vi "Values.vi"(8 "error in (no error)":errorcluster, 11 "VariantAttribute in":refnum<class "MapImp.lvclass">) -> (0 "error out":errorcluster, 1 "Values":refnum<class>[](array[class]), 3 "VariantAttribute out":refnum<class "MapImp.lvclass">)   [LabVIEW 2013, in "LapDog.Collections.v_.Maps.lvlib" / "MapImp.lvclass"]
doc: "Returns a copy of all values in the map."
uses:
  MapImp.lvclass
  MapImp.lvclass/MapImp.ctl
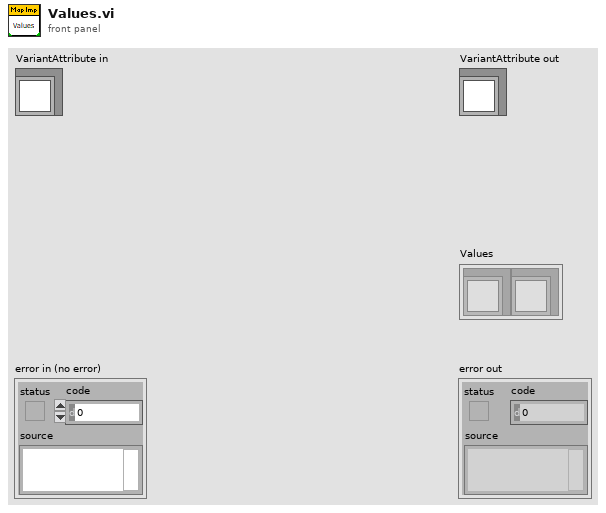
[diagram p1: front panel]
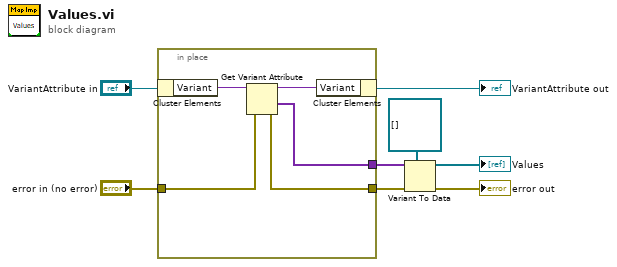
[diagram p0: block diagram]
diagram:
  n1 = in-place {
    in-place-border: "error in (no error)" -> [w12]
    in-place-border: [w11] -> w4
    in-place-border: [w9] -> w3
    n2 = in-place-cluster #1("VariantAttribute in") -> ("Variant"=w13:variant)
    n3 = Get Variant Attribute(Variant=w13, error in=w12) -> (duplicate Variant=w10:variant, values=w9:variant[], error out=w11:errorcluster)  [unwired: 2 in, 1 out]
    n4 = in-place-cluster #1("Variant"=w10) -> (→"VariantAttribute out":refnum<class "MapImp.lvclass">)
  }
  n5 = Variant To Data(error in=w4, type=refnum<class>[] [], Variant=w3) -> (data=→"Values":refnum<class>[], error out=→"error out":errorcluster)
